vi "Flush Exit.vi"(8 "error in (no error)":errorcluster, 11 "Data":variant) -> (0 "error out":errorcluster)   [LabVIEW 2014, in "Controller (Host).lvlib"]
doc: "This subVI enqueues the Exit action in to the communications queue along with the input data after flushing the queue."
uses:
  Controller (Host).lvlib
  Private Controls/Module Data.ctl
  Private Controls/Module Action.ctl
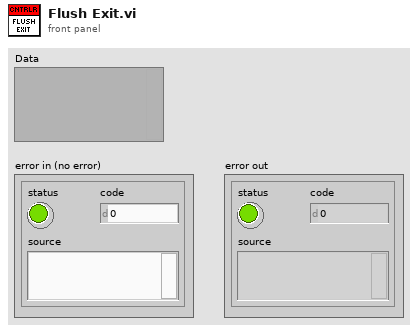
[diagram p1: front panel]
types:
  T1 = typedef "Controller (Host).lvlib/Module Data.ctl" = cluster{"Data":variant, "Action":T2}
  T2 = typedef "Controller (Host).lvlib/Module Action.ctl" = enum8{"Timeout", "Init", "Error", "Exit", "Set cRIO Connected Status", "Prompt Login", "Prompt Main Menu", "Prompt APU Select", "Prompt Operation Select", "Prompt SubTests Select", "Prompt Break Out", "Calibration", "Testing", "Load User Info", "Set Instr Init Status", "Load APU Setup Data", "Engine Start Val Change", "RPM Cross 95Perc Thresh", "Interactive Ctrls Val Change"}
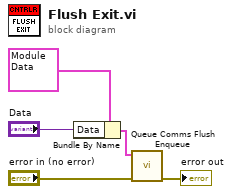
[diagram p0: block diagram]
diagram:
  n1 = Bundle By Name(cluster=T1 {"Data"=variant, "Action"=enum."Exit"} ("element"), "Data"="Data") -> (w1:T1)
  n2 = call "Queue Comms Flush Enqueue.vi"("error in (no error)"="error in (no error)", "element"=w1) -> ("error out"=→"error out":errorcluster)  [unwired: 9 in]
